vi "read.vi"(8 "error in (no error)":errorcluster, 10 "Command":string="I_C_1:A_C?", 11 "NEXUS in":refnum<class "NEXUS.lvclass">) -> (0 "error out":errorcluster, 2 "Response":string, 3 "NEXUS out":refnum<class "NEXUS.lvclass">)   [LabVIEW 2019, in "NEXUS.lvclass"]
uses:
  NEXUS.lvclass
  <vilib>/Instr/_visa.llb/VISA Configure Serial Port (Instr).vi
panel:
  in  "Read Count":u32=1000
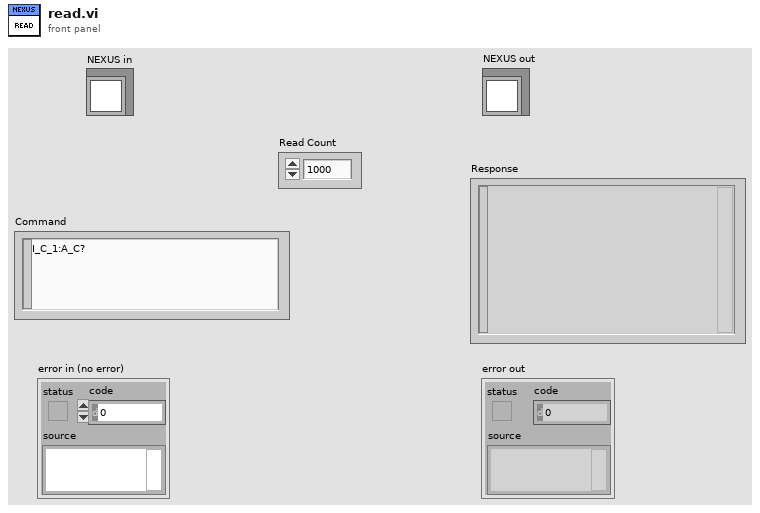
[diagram p1: front panel]
types:
  T1 = cluster{"baud rate":u32, "data bits":u16, "parity":enum16{"None", "Odd", "Even", "Mark", "Space"}, "stop bits":u16, "flow control":u16}
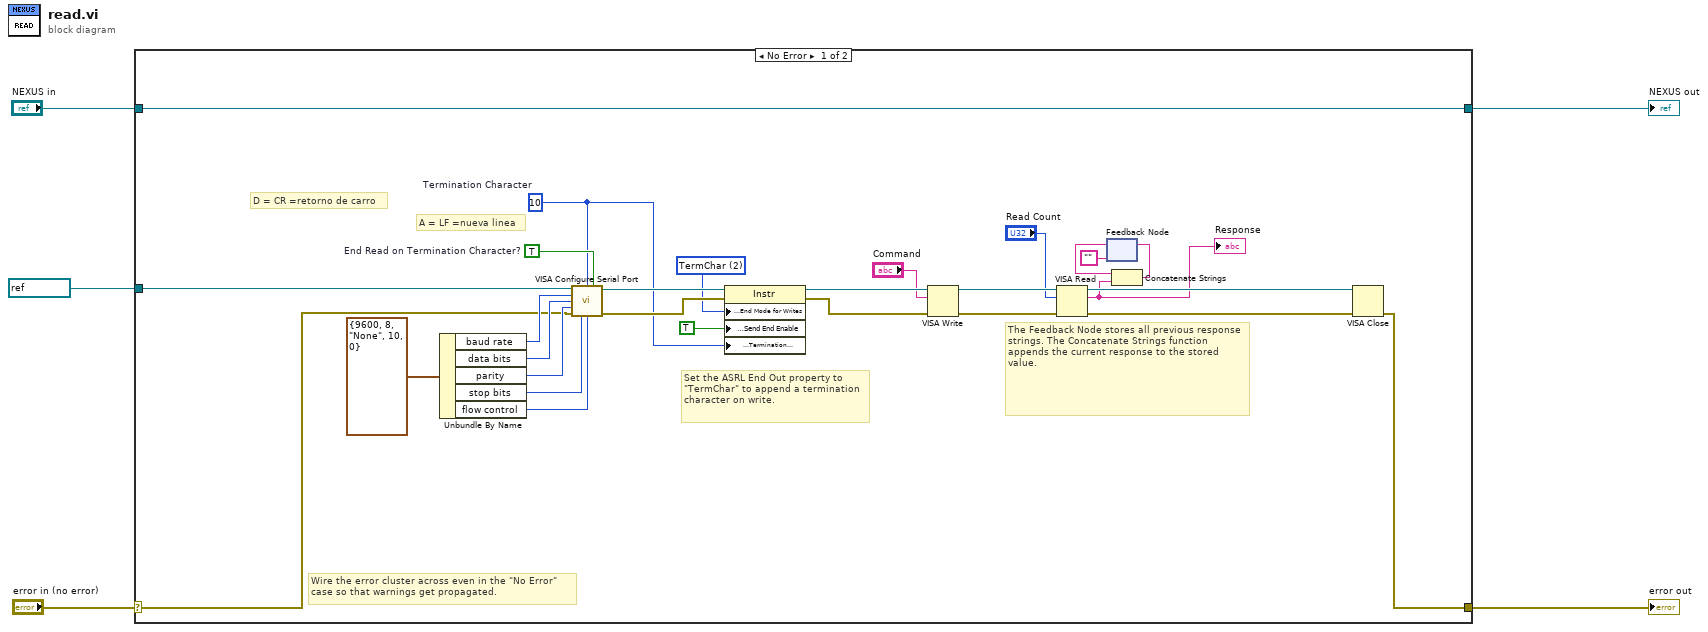
[diagram p0: block diagram]
diagram:
  n1 = case shown="No Error" "error in (no error)" {
    selector: "error in (no error)" -> [w12 w35]
    tunnel: [w11 w35] -> w4
    tunnel: [w33 w34] -> w2
    tunnel: "NEXUS in" -> [w33 w34]
    tunnel: refnum<visa-resource-name> "COM6" ("VISA resource name") -> [w13 _]
    frame No Error {
      w15 = u16 2 items=["None", "LastBit", "TermChar", "Break"] ("Serial Settings:Serial End Mode for Writes")
      w19 = u8 10  # Termination Character
      w25 = TRUE  # End Read on Termination Character?
      # "The Feedback Node stores all previous response strings. The Concatenate Strings function appends the current response to the stored value."
      # "Set the ASRL End Out property to \"TermChar\" to append a termination character on write."
      # "D = CR =retorno de carro"
      # "A = LF =nueva linea"
      # "Wire the error cluster across even in the \"No Error\"\ncase so that warnings get propagated."
      n2 = Unbundle By Name(T1 {"baud rate"=9600, "data bits"=8, "parity"=enum."None", "stop bits"=10, "flow control"=0} ("Serial Settings")) -> ("baud rate"=w27:u32, "data bits"=w28:u16, "parity"=w29:enum16{"None", "Odd", "Even", "Mark", "Space"}, "stop bits"=w30:u16, "flow control"=w22:u16)
      n3 = call-poly "VISA Configure Serial Port"("VISA resource name"=w13, "termination char\n(0xA = '\\n' = LF)"=w19, "Enable Termination\nChar (T)"=w25, "baud rate (9600)"=w27, "data bits (8)"=w28, "parity (0:none)"=w29, "error in (no error)"=w12, "stop bits (10: 1 bit)"=w30, "flow control (0:none)"=w22) -> ("VISA resource name out"=w31:refnum<visa-resource-name>, "error out"=w32:errorcluster)  [unwired: 1 in, 4 out]
      n4 = property class="Instr"(reference=w31, error in=w32, "Serial Settings:End Mode for Writes"=w15, "Message Based Settings:Send End Enable"=TRUE, "Message Based Settings:Termination Character"=w19) -> (reference out=w20:refnum<visa-resource-name>, error out=w21:errorcluster)
      n5 = VISA Write(VISA resource name=w20, write buffer="Command", error in (no error)=w21) -> (VISA resource name out=w18:refnum<visa-resource-name>, error out=w17:errorcluster)  [unwired: 1 out]
      n6 = VISA Read(VISA resource name=w18, byte count="Read Count", error in (no error)=w17) -> (VISA resource name out=w23:refnum<visa-resource-name>, read buffer=w6:string, error out=w24:errorcluster)  [unwired: 1 out]
      "Response" <- w6
      n7 = feedback #1("") -> (w9:string)
      n8 = Concatenate Strings(w9, w6) -> (w8:string)
      n9 = feedback-in #1(w8) -> ()
      n10 = VISA Close(VISA resource name=w23, error in (no error)=w24) -> (error out=w11:errorcluster)
    }
    frame Error {
    }
  }
  "error out" <- w4
  "NEXUS out" <- w2
